vi "Create.vi"(8 "error in (no error)":errorcluster, 10 "String":string) -> (0 "error out":errorcluster, 3 "Words to Numbers Converter":refnum<class "Words to Numbers Converter.lvclass">)   [LabVIEW 2020, in "Words to Numbers Converter.lvclass"]
uses:
  Words to Numbers Converter.lvclass
  Words to Numbers Converter.lvclass/Words to Numbers Converter.ctl
  bb65fb00-7284-4297-a26c-1f0a0fc059be.vi
  <vilib>/Comparison/Less/Less Functor/Less Functor.lvclass
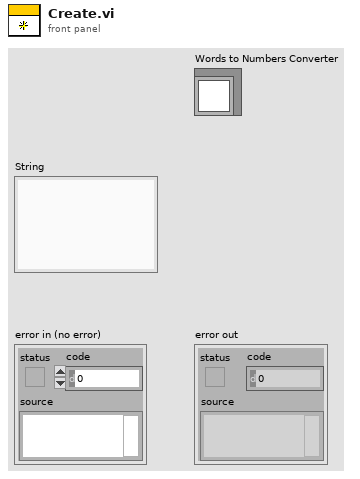
[diagram p1: front panel]
types:
  T1 = typedef "Words to Numbers Converter.lvclass/Word in String.ctl" = cluster{"Offset":i32, "Word":string, "numeric value":i32}
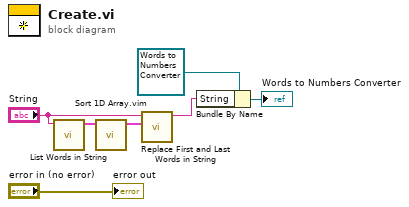
[diagram p0: block diagram]
diagram:
  n1 = call "List Words in String.vi"("String"="String") -> ("Array"=w4:T1[])  [unwired: 10 in]
  n2 = call "Sort 1D Array.vim"("unsorted array"=w4) -> ("sorted array"=w3:T1[])  [unwired: 10 in]
  n3 = call "Replace First and Last Words in String.vi"("sorted array"=w3, "String in"="String") -> ("String out"=w2:string)  [unwired: 9 in]
  n4 = Bundle By Name(cluster=refnum<class "Words to Numbers Converter.lvclass"> refnum ("Words to Numbers Converter"), "String"=w2) -> (→"Words to Numbers Converter":refnum<class "Words to Numbers Converter.lvclass">)
  "error out" <- "error in (no error)"
